vi "GetLowlevelParas_KCubeDCServo.vi"(11 ".NET Refnum in":refnum<k24>) -> (1 "Cluster 2":T2, 2 "Cluster":cluster{"Acceleration":dbl, "MaxVelocity":dbl}, 3 "Cluster 3":T1)   [LabVIEW 2019]
doc: "get low-level parameters (velocity and acceleration) for DC servo motors."
uses:
  D:/Victor Sun/optical trap control/Kinesis/ThorLabs.MotionControl.KCube.DCServoCLI.dll
  Kinesis/ThorLabs.MotionControl.KCube.DCServoCLI.dll
  D:/Victor Sun/optical trap control/Kinesis/Thorlabs.MotionControl.GenericMotorCLI.dll
  Kinesis/Thorlabs.MotionControl.GenericMotorCLI.dll
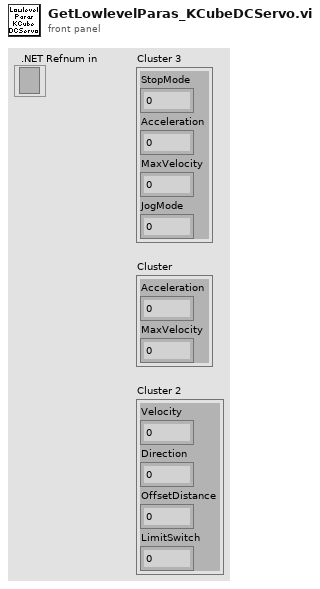
[diagram p1: front panel]
types:
  T1 = cluster{"StopMode":i16, "Acceleration":dbl, "MaxVelocity":dbl, "JogMode":i16}
  T2 = cluster{"Velocity":dbl, "Direction":i32, "OffsetDistance":dbl, "LimitSwitch":i32}
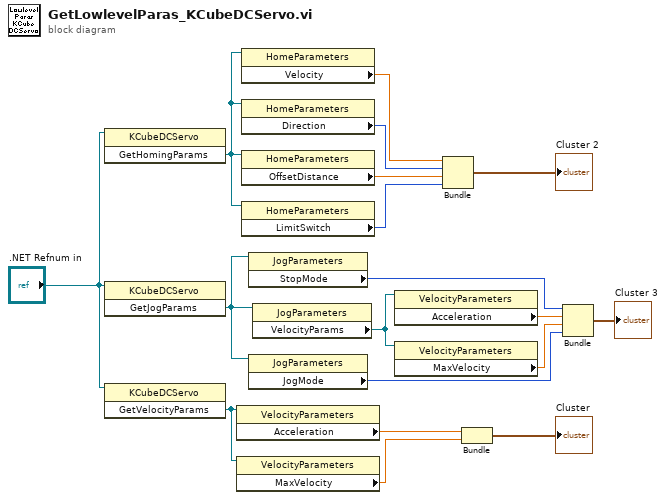
[diagram p0: block diagram]
diagram:
  n1 = invoke class="KCubeDCServo" method="GetHomingParams"(reference=".NET Refnum in") -> ("GetHomingParams"=w4:refnum<k24>)  [unwired: 2 in, 2 out]
  n2 = invoke class="KCubeDCServo" method="GetJogParams"(reference=".NET Refnum in") -> ("GetJogParams"=w2:refnum<k24>)  [unwired: 2 in, 2 out]
  n3 = invoke class="KCubeDCServo" method="GetVelocityParams"(reference=".NET Refnum in") -> ("GetVelocityParams"=w3:refnum<k24>)  [unwired: 2 in, 2 out]
  n4 = property class="VelocityParameters"(reference=w3) -> ("Acceleration"=w16:dbl)  [unwired: 1 in, 2 out]
  n5 = property class="VelocityParameters"(reference=w3) -> ("MaxVelocity"=w17:dbl)  [unwired: 1 in, 2 out]
  n6 = property class="HomeParameters"(reference=w4) -> ("Velocity"=w12:dbl)  [unwired: 1 in, 2 out]
  n7 = property class="HomeParameters"(reference=w4) -> ("Direction"=w13:i32)  [unwired: 1 in, 2 out]
  n8 = property class="HomeParameters"(reference=w4) -> ("OffsetDistance"=w14:dbl)  [unwired: 1 in, 2 out]
  n9 = property class="HomeParameters"(reference=w4) -> ("LimitSwitch"=w15:i32)  [unwired: 1 in, 2 out]
  n10 = property class="JogParameters"(reference=w2) -> ("StopMode"=w6:i16)  [unwired: 1 in, 2 out]
  n11 = property class="JogParameters"(reference=w2) -> ("JogMode"=w9:i16)  [unwired: 1 in, 2 out]
  n12 = property class="JogParameters"(reference=w2) -> ("VelocityParams"=w1:refnum<k24>)  [unwired: 1 in, 2 out]
  n13 = property class="VelocityParameters"(reference=w1) -> ("Acceleration"=w7:dbl)  [unwired: 1 in, 2 out]
  n14 = property class="VelocityParameters"(reference=w1) -> ("MaxVelocity"=w8:dbl)  [unwired: 1 in, 2 out]
  n15 = Bundle("Velocity"=w12, "Direction"=w13, "OffsetDistance"=w14, "LimitSwitch"=w15) -> (→"Cluster 2":T2)  [unwired: 1 in]
  n16 = Bundle("Acceleration"=w16, "MaxVelocity"=w17) -> (→"Cluster":cluster{"Acceleration":dbl, "MaxVelocity":dbl})  [unwired: 1 in]
  n17 = Bundle("StopMode"=w6, "Acceleration"=w7, "MaxVelocity"=w8, "JogMode"=w9) -> (→"Cluster 3":T1)  [unwired: 1 in]
